vi "dfd_Super Narrowband Filter Design Call Old Method.vi"(6 "ripple specs":T1={"passband"=0.05, "stopband"=60.0, "dB/linear? (T: dB)"=TRUE}, 7 "filter type":T2(ring), 8 "error in (no error)":errorcluster, 9 "fc":dbl, 10 "fstop":dbl, 11 "fpass":dbl) -> (0 "error out":errorcluster, 2 "new filter type":T8(ring), 3 "multirate filters out":T3[](array[typedef]) {"mMRate_SumWl" min=1 max=32 step=1; "mMRate_InputIwl" min=1 max=32 step=1; "mMRate_GainWl" min=1 max=32 step=1; "mMRate_OutputWl" min=1 max=32 step=1; "mMRate_InputWl" min=1 max=32 step=1; "mMRate_CoefWl" min=1 max=32 step=1; "mMRate_Mode" items=["Default"=-1, "No Rate Change"=0, "Interpolation"=1, "Decimation"=2, "Interpolated"=3, "Rational"=4]})   [LabVIEW 2017, in "NI_DigFilter_Process.lvlib"]
uses:
  <vilib>/addons/Digital Filter Design/NI_DigFilter_Process.lvlib
  <vilib>/addons/Digital Filter Design/_Objects.llb/DFD Multirate Filter Obj.ctl
  <vilib>/addons/Digital Filter Design/_Objects.llb/DFD Multirate Mode.ctl
  <vilib>/addons/Digital Filter Design/_Objects.llb/DFD Coef Norm Type.ctl
  <vilib>/addons/Digital Filter Design/_Objects.llb/DFD Round-off Mode.ctl
  <vilib>/addons/Digital Filter Design/_Objects.llb/DFD FXP MRate Multiply Mode.ctl
  <vilib>/addons/Digital Filter Design/_Objects.llb/DFD Filter Ripple Specification (Design).ctl
  <vilib>/Analysis/NI_AALBase.lvlib
  <vilib>/addons/Digital Filter Design/NI_DigFilter_Design.lvlib
  <vilib>/addons/Digital Filter Design/NI_DigFilterLicensed.lvlib
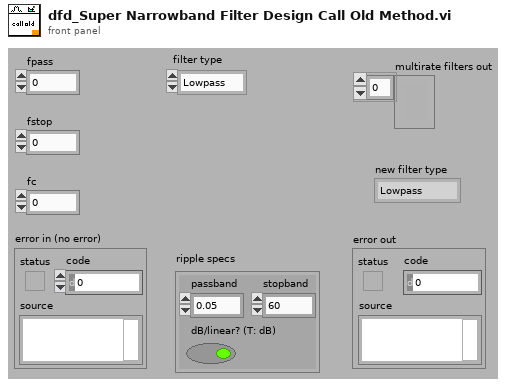
[diagram p1: front panel]
types:
  T1 = typedef "NI_DigFilterLicensed.lvlib/DFD Filter Ripple Specification (Design).ctl" = cluster{"passband":dbl, "stopband":dbl, "dB/linear? (T: dB)":bool}
  T2 = enum16{"Lowpass", "Highpass", "Bandpass", "Bandstop"}
  T3 = typedef "NI_DigFilterLicensed.lvlib/DFD Multirate Filter Obj.ctl" = cluster{"mMRate_Structure":enum16{"CIC", "FIR", "IIR", "Lattice"}, "mMRate_Mode":T4, "mMRate_Factor":i32, "mMRate_FIRParams":cluster{"mMRate_FIR_H":dbl[], "mMRate_FIR_IsNyquist?":bool, "mMRate_FIR_IsSymmetric?":bool}, "mMRate_CICParams":cluster{"mMRate_CIC_#Stage":i32, "mMRate_CIC_Lag":i32, "mMRate_CIC_Type":enum16{"Lowpass", "Highpass"}}, "mMRate_Order":i32, "mMRate_Version":string, "mMRate_Comments":string, "mMRate_RationalFactor":cluster{"mMRate_L":i32, "mMRate_M":i32}, "mMRate_Fs":dbl, "mMRate_Quantized?":bool, "mMRate_QFilterGain":dbl, "mMRate_CoefWl":i16, "mMRate_Scaling":cluster{"mMRate_ScaleByPowerOf2?":bool, "mMRate_ScaleType":T5}, "mMRate_InputWl":i16, "mMRate_OutputWl":i16, "mMRate_OutputMode":T6, "mMRate_MultMode":T7, "mMRate_BitPruning":bool, "mMRate_GainWl":i16, "mMRate_OutputFwl":i16, "mMRate_SumIwl":i16, "mMRate_InputIwl ":i16, "mMRate_SumWl":i16, "mMRate_CoefIwl":i16}
  T4 = typedef "NI_DigFilterLicensed.lvlib/DFD Multirate Mode.ctl" = i16
  T5 = typedef "NI_DigFilterLicensed.lvlib/DFD Coef Norm Type.ctl" = enum16{"No Norm", "Time Domain 1-Norm", "Time Domain 2-Norm", "Time Domain Inf-Norm"}
  T6 = typedef "NI_DigFilterLicensed.lvlib/DFD Round-off Mode.ctl" = enum16{"Nearest", "Truncation"}
  T7 = typedef "NI_DigFilterLicensed.lvlib/DFD FXP MRate Multiply Mode.ctl" = enum16{"Truncated", "Full"}
  T8 = enum32{"Lowpass", "Highpass", "Bandpass", "Bandstop", "Wideband-Lowpass", "Wideband-Highpass"}
  T9 = cluster{"filter type":enum32{"Lowpass", "Highpass", "Bandpass", "Bandstop", "Wideband-Lowpass", "Wideband-Highpass"}, "interpolation":i32, "Model Filter":dbl[], "Image Suppressor":dbl[]}
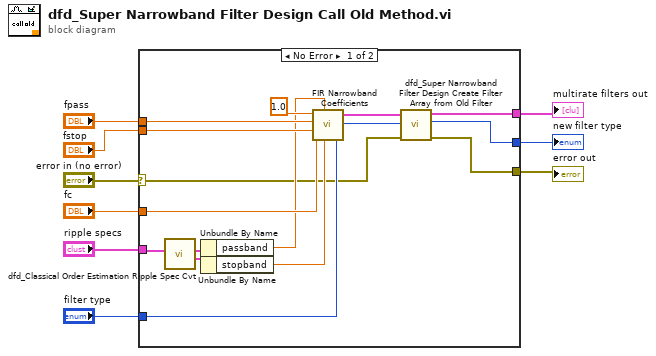
[diagram p0: block diagram]
diagram:
  n1 = case shown="No Error" "error in (no error)" {
    selector: "error in (no error)" -> [w10 w26]
    tunnel: [w12 _] -> w9
    tunnel: [w24 w26] -> w8
    tunnel: [w23 _] -> w7
    tunnel: "fstop" -> [w22 _]
    tunnel: "fpass" -> [w21 _]
    tunnel: "fc" -> [w20 _]
    tunnel: "filter type" -> [w19 _]
    tunnel: "ripple specs" -> [w17 _]
    frame No Error {
      n2 = call <vilib>:"dfd_Classical Order Estimation Ripple Spec Cvt.vi"("ripple specs"=w17) -> ("ripple specs (dB)"=w14:T1, "ripple specs (linear)"=w16:T1)  [unwired: 9 out]
      n3 = Unbundle By Name(w16) -> ("passband"=w15:dbl)
      n4 = Unbundle By Name(w14) -> ("stopband"=w13:dbl)
      n5 = call <vilib>:"FIR Narrowband Coefficients.vi"("sampling freq: fs"=1.0, "ripple: rp"=w15, "passband: fpass"=w21, "stopband: fstop"=w22, "attenuation (db): Ar"=w13, "center freq: fc"=w20, "filter type"=w19) -> ("IFIR Coefficients"=w25:T9, "error"=w11:i32)
      n6 = call <vilib>:"dfd_Super Narrowband Filter Design Create Filter Array from Old Filter.vi"("error in (no error)"=w10, "error"=w11, "IFIR Coefficients"=w25) -> ("error out"=w24:errorcluster, "new filter type"=w12:T8, "multirate filters out"=w23:T3[])  [unwired: 6 out]
    }
    frame Error {
    }
  }
  "new filter type" <- w9
  "error out" <- w8
  "multirate filters out" <- w7
